vi "Test Find Leaks.vi"(4 "error in":errorcluster) -> (0 "error out":errorcluster)   [LabVIEW 2025]
doc: "Unit Test for <i>Find Leaks.vi</i>. This test generates all VIs and projects according to the definition files, exports the strings and searches for leaks with the VI-under-test. \n\nThe test checks finding of secrets and error generation in a clean and a dirty project."
uses:
  src/Type Definitions/Secret--cluster.ctl
  src/Type Definitions/Leak--cluster.ctl
  <vilib>/addons/_JKI Toolkits/Caraya/classes/Assert/Assert Not Error.vi
  <vilib>/addons/_JKI Toolkits/Caraya/classes/Assert/Assert True.vi
  <vilib>/addons/_JKI Toolkits/Caraya/classes/Assert/Assert Error.vi
  <vilib>/regexp/Match Regular Expression.xnode
  <vilib>/addons/_JKI Toolkits/Caraya/classes/Assert/Assert.lvclass
  <vilib>/addons/_JKI Toolkits/Caraya/classes/Test/Test.lvclass
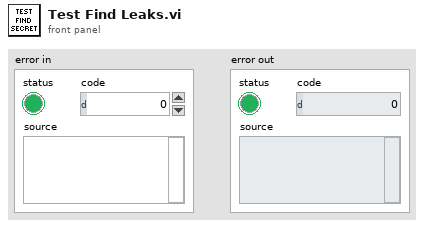
[diagram p1: front panel]
types:
  T1 = typedef "Leak--cluster.ctl" = cluster{"Secret":T2, "Value":string}
  T2 = typedef "Secret--cluster.ctl" = cluster{"Name":string, "Regex":string}
  T3 = typedef "Element Strings--cluster.ctl" = cluster{"Element Name":string, "Strings":string[]}
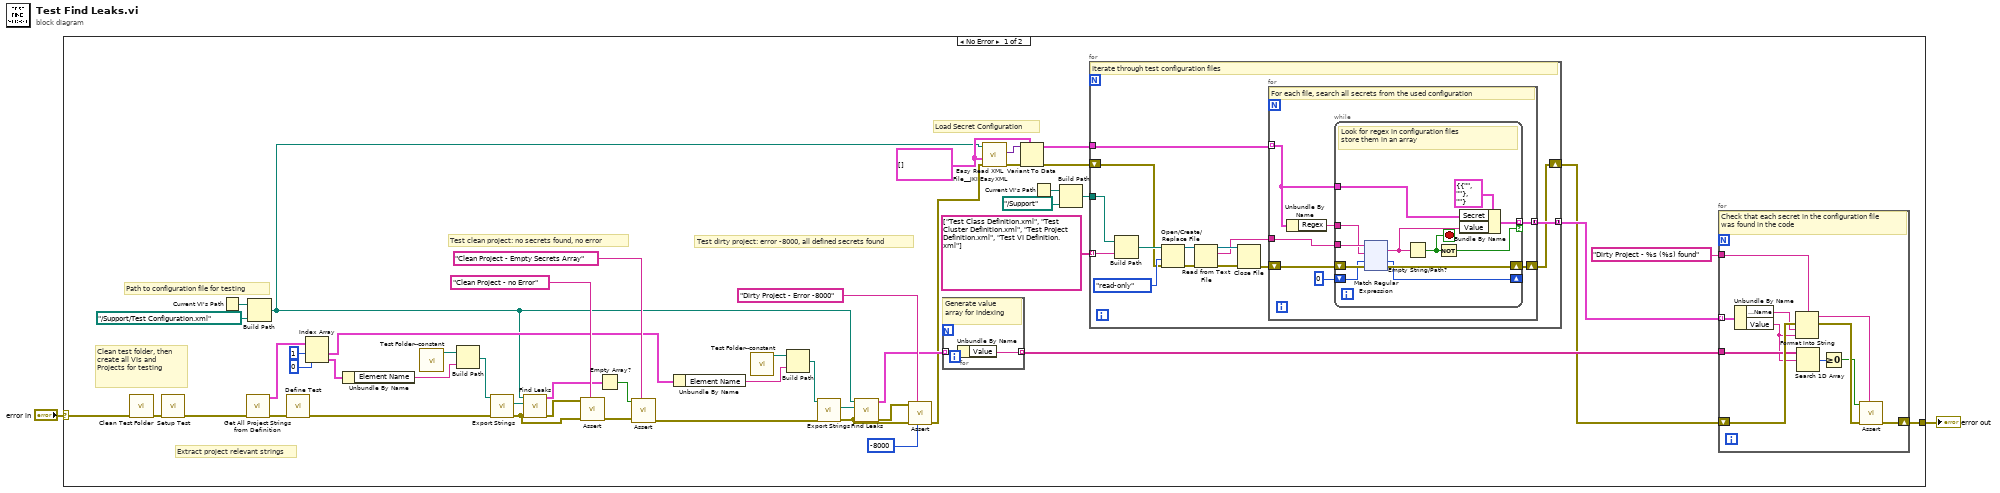
[diagram p0: block diagram]
diagram:
  n1 = case shown="No Error" "error in" {
    selector: "error in" -> [w41 w215]
    tunnel: [w42 w215] -> w1
    frame No Error {
      w9 = T2[] [] ("Array")
      # "Load Secret Configuration"
      # "Test dirty project: error -8000, all defined secrets found"
      # "Test clean project: no secrets found, no error"
      # "Extract project relevant strings"
      # "Path to configuration file for testing"
      # "Clean test folder, then create all VIs and\nProjects for testing"
      n2 = call "Clean Test Folder.vi"("error in"=w41) -> ("error out"=w51:errorcluster)  [unwired: 6 in]
      n3 = call "Setup Test.vi"("error in"=w51) -> ("error out"=w40:errorcluster)  [unwired: 6 in]
      n4 = Current VI's Path() -> (path=w33:path)
      n5 = call "Get All Project Strings from Definition.vi"("error in"=w40) -> ("error out"=w49:errorcluster, "Project Strings"=w36:T3[])  [unwired: 5 in]
      n6 = Build Path(base path=w33, name or relative path=path "../Support/Test Configuration.xml") -> (appended path=w8:path)
      n7 = call <vilib>:"Define Test.vi"("error in (no error)"=w49) -> ("error out"=w50:errorcluster)  [unwired: 9 in, 1 out]
      n8 = Index Array(array=w36, index #1=1 ("index"), index #2=0 ("index")) -> (element #1=w20:T3, element #2=w26:T3)
      n9 = Unbundle By Name(w26) -> ("Element Name"=w37:string)
      n10 = call "Test Folder--constant.vi"() -> ("Test Folder"=w39:path)  [unwired: 7 in]
      n11 = Build Path(base path=w39, name or relative path=w37) -> (appended path=w38:path)
      n12 = call "Export Strings.vi"("error in"=w50, "Target"=w38) -> ("error out"=w48:errorcluster, "String File Out"=w34:path)  [unwired: 3 in, 1 out]
      n13 = call "Find Leaks.vi"("error in"=w48, "String File"=w34, "Secrets Configuration"=w8) -> ("error out"=w47:errorcluster, "Leaks"=w29:T1[])  [unwired: 2 in, 1 out]
      n14 = call-poly <vilib>:"Assert.vi"("Label"="Clean Project - no Error", "error in (no error)"=w48, "Not Error?"=w47) -> ("error out"=w46:errorcluster)  [unwired: 7 in, 1 out]
      n15 = Empty Array?(array=w29) -> (empty?=w28:bool)
      n16 = call-poly <vilib>:"Assert.vi"("Label"="Clean Project - Empty Secrets Array", "error in (no error)"=w46, "True?"=w28) -> ("error out"=w43:errorcluster)  [unwired: 7 in, 1 out]
      n17 = Unbundle By Name(w20) -> ("Element Name"=w23:string)
      n18 = call "Test Folder--constant.vi"() -> ("Test Folder"=w25:path)  [unwired: 7 in]
      n19 = Build Path(base path=w25, name or relative path=w23) -> (appended path=w24:path)
      n20 = call "Export Strings.vi"("error in"=w43, "Target"=w24) -> ("error out"=w45:errorcluster, "String File Out"=w22:path)  [unwired: 3 in, 1 out]
      n21 = call "Find Leaks.vi"("error in"=w45, "String File"=w22, "Secrets Configuration"=w8) -> ("error out"=w44:errorcluster, "Leaks"=w18:T1[])  [unwired: 2 in, 1 out]
      n22 = call-poly <vilib>:"Assert.vi"("error code (1)"=-8000, "Label"="Dirty Project - Error -8000", "error in (no error)"=w45, "Error?"=w44) -> ("error out"=w4:errorcluster)  [unwired: 6 in, 1 out]
      n23 = for {
        tunnel: w18 -> [w214] mode=indexing
        tunnel: [w213] -> w16 mode=indexing
        # "Generate value array for indexing"
        n24 = Unbundle By Name(w214) -> ("Value"=w213:string)
      }
      n25 = call <vilib>:"Easy Read XML File__JKI EasyXML.vi"("error in (no error)"=w4, "LabVIEW Data (Type)"=w9, "XML File Path"=w8) -> ("error out"=w11:errorcluster, "LabVIEW Data"=w10:variant)  [unwired: 6 in, 1 out]
      n26 = Variant To Data(error in=w11, type=w9, Variant=w10) -> (data=w6:T2[], error out=w7:errorcluster)
      n27 = Current VI's Path() -> (path=w15:path)
      n28 = Build Path(base path=w15, name or relative path=path "../Support") -> (appended path=w12:path)
      n29 = for {
        tunnel: string[] ["Test Class Definition.xml", "Test Cluster Definition.xml", "Test Project Definition.xml", "Test VI Definition.xml"] -> [w64] mode=indexing
        tunnel: w12 -> [w65]
        shift-right: [w52] -> w3
        shift-left: w7 -> [w54]
        tunnel: w6 -> [w55]
        tunnel: [w53] -> w5 mode=concatenating
        # "Iterate through test configuration files"
        n30 = Build Path(base path=w65, name or relative path=w64) -> (appended path=w63:path)
        n31 = Open/Create/Replace File(file path (use dialog)=w63, error in=w54, access (0:read/write)=enum16{"read/write", "read-only", "write-only"}."read-only") -> (refnum out=w60:refnum<file>, error out=w61:errorcluster)  [unwired: 3 in, 1 out]
        n32 = Read from Text File(file (use dialog)=w60, error in=w61) -> (refnum out=w58:refnum<file>, text=w57:string, error out=w59:errorcluster)  [unwired: 2 in, 1 out]
        n33 = Close File(refnum=w58, error in=w59) -> (error out=w56:errorcluster)  [unwired: 1 out]
        n34 = for {
          tunnel: w57 -> [w68]
          tunnel: w55 -> [w69] mode=indexing
          shift-right: [w66] -> w52
          shift-left: w56 -> [w71]
          tunnel: [w67] -> w53 mode=concatenating
          # "For each file, search all secrets from the used configuration"
          n35 = Unbundle By Name(w69) -> ("Regex"=w70:string)
          n36 = while {
            tunnel: w68 -> [w84]
            tunnel: w70 -> [w83]
            shift-right: [w81] -> w66
            shift-left: w71 -> [w82]
            shift-right: [w79] -> _
            shift-left: 0 -> [w80]
            tunnel: [w75] -> w67 mode=indexing if=w78
            tunnel: w69 -> [w76]
            stop <- w73 stop-if-true
            # "Look for regex in configuration files\nstore them in an array"
            n37 = xnode "Match Regular Expression"("input string"=w84, "regular expression"=w83, "offset (0)"=w80, "error in"=w82) -> ("whole match"=w74:string, "offset past match"=w79:i32, "error out"=w81:errorcluster)  [unwired: 2 in, 2 out]
            n38 = Empty String/Path?(string/path=w74) -> (empty?=w73:bool)
            n39 = Not(x=w73) -> (.not. x?=w78:bool)
            n40 = Bundle By Name(cluster=T1 {"Secret"={"Name"="", "Regex"=""}, "Value"=""} ("Leak"), "Secret"=w76, "Value"=w74) -> (w75:T1)
          }
        }
      }
      n41 = for {
        tunnel: "Dirty Project - %s (%s) found" ("format string") -> [w209]
        tunnel: w5 -> [w204] mode=indexing
        tunnel: w16 -> [w208]
        shift-right: [w212] -> w42
        shift-left: w3 -> [w211]
        # "Check that each secret in the configuration file\nwas found in the code"
        n42 = Unbundle By Name(w204) -> ("Secret.Name"=w203:string, "Value"=w202:string)
        n43 = Format Into String(format string=w209, error in=w211, w203, w202) -> (resulting string=w206:string, error out=w210:errorcluster)  [unwired: 1 in]
        n44 = Search 1D Array(1D array=w208, element=w202) -> (index of element=w207:i32)  [unwired: 1 in]
        n45 = Greater Or Equal To 0?(x=w207) -> (x >= 0?=w205:bool)
        n46 = call-poly <vilib>:"Assert.vi"("Label"=w206, "error in (no error)"=w210, "True?"=w205) -> ("error out"=w212:errorcluster)  [unwired: 7 in, 1 out]
      }
    }
    frame Error {
      # "Pass error without further action"
    }
  }
  "error out" <- w1
